vi "RemoveFirstElement.vi"(6 "Delays12 in":dbl[](array[numeric]), 7 "Second It?":bool, 8 "Three Events In":dbl[][](array[numeric]), 9 "Two Events In":dbl[][](array[numeric]), 10 "Delays02 in":dbl[](array[numeric]), 11 "Delays01 in":dbl[](array[numeric])) -> (0 "Three Events out":dbl[][](array[numeric]), 1 "Two Events Out":dbl[][](array[numeric]), 2 "Delays02 out":dbl[](array[numeric]), 3 "Delays01 out":dbl[](array[numeric]), 4 "Delays12 out":dbl[](array[numeric]))   [LabVIEW 2023]
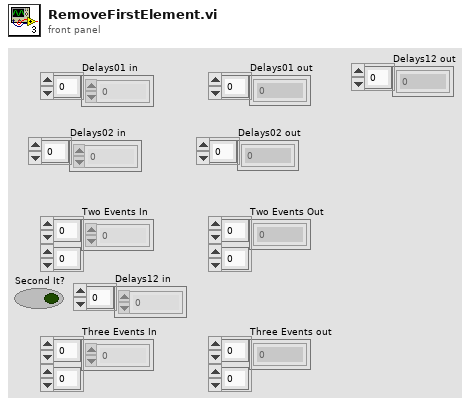
[diagram p1: front panel]
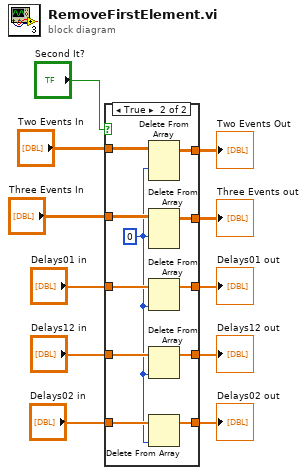
[diagram p0: block diagram]
diagram:
  n1 = case shown="True" "Second It?" {
    tunnel: "Three Events In" -> [w16 w27]
    tunnel: [w16 w26] -> w7
    tunnel: "Two Events In" -> [w15 w25]
    tunnel: [w15 w24] -> w9
    tunnel: "Delays01 in" -> [w14 w22]
    tunnel: [w14 w23] -> w11
    tunnel: "Delays02 in" -> [w13 w21]
    tunnel: [w13 w20] -> w3
    tunnel: "Delays12 in" -> [w12 w19]
    tunnel: [w12 w18] -> w1
    frame False {
    }
    frame True {
      w17 = 0 ("index (row)")
      n2 = Delete From Array(array=w25, index (row)=w17) -> (array with subset deleted=w24:dbl[][])  [unwired: 2 in, 1 out]
      n3 = Delete From Array(array=w27, index (row)=w17) -> (array with subset deleted=w26:dbl[][])  [unwired: 2 in, 1 out]
      n4 = Delete From Array(array=w22, index=w17) -> (array with subset deleted=w23:dbl[])  [unwired: 1 in, 1 out]
      n5 = Delete From Array(array=w19, index=w17) -> (array with subset deleted=w18:dbl[])  [unwired: 1 in, 1 out]
      n6 = Delete From Array(array=w21, index=w17) -> (array with subset deleted=w20:dbl[])  [unwired: 1 in, 1 out]
    }
  }
  "Delays01 out" <- w11
  "Two Events Out" <- w9
  "Three Events out" <- w7
  "Delays02 out" <- w3
  "Delays12 out" <- w1
